vi "Default Settings.vi"() -> (3 "Default Settings":T1={"Log File Base Path"=path "", "Analog Input Channel"="", "Max Value"=0.0, "Min Value"=-5.0})   [LabVIEW 2020, in "Settings Editor.lvlib"]
doc: "_____\nBased on Delacor QMH Project Template 5.0.0.82."
uses:
  Settings Editor.lvlib
  Settings--cluster.ctl
  <vilib>/Utility/sysdir.llb/System Directory Type.ctl
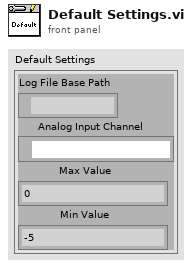
[diagram p1: front panel]
types:
  T1 = typedef "Settings Editor.lvlib/Settings--cluster.ctl" = cluster{"Log File Base Path":path, "Analog Input Channel":refnum<k21>, "Max Value":dbl, "Min Value":dbl}
  T2 = typedef "System Directory Type.ctl" = i32
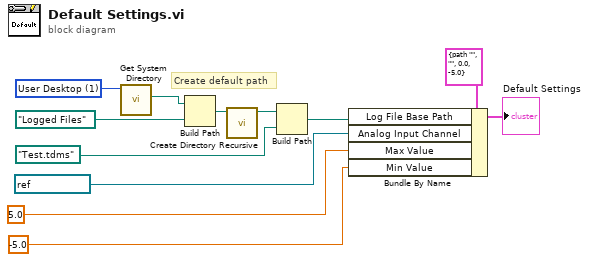
[diagram p0: block diagram]
diagram:
  w12 = T2 1 items=["User Home"=0, "User Desktop"=1, "User Documents"=2, "User Application Data"=3, "User Preferences"=4, "User Temporary"=5, "Public Documents"=6, "Public Application Data"=7, "Public Preferences"=8, "Public Cache"=13, "System Core Libraries"=9, "System Installed Libraries"=10, "Application Files"=11, "Boot Volume Root"=12] ("system directory type")
  # "Create default path"
  n1 = call <vilib>:"Get System Directory.vi"("system directory type"=w12) -> ("system directory"=w11:path)  [unwired: 10 in]
  n2 = Build Path(base path=w11, name or relative path=path "Logged Files") -> (appended path=w10:path)
  n3 = call <vilib>:"Create Directory Recursive.vi"("directory"=w10) -> ("directory copy"=w9:path)  [unwired: 4 in, 2 out]
  n4 = Build Path(base path=w9, name or relative path=path "Test.tdms") -> (appended path=w6:path)
  n5 = Bundle By Name(cluster=T1 {"Log File Base Path"=path "", "Analog Input Channel"="", "Max Value"=0.0, "Min Value"=-5.0} ("Default Settings"), "Log File Base Path"=w6, "Analog Input Channel"=refnum<k21> "Dev0/Ai0", "Max Value"=5.0, "Min Value"=-5.0) -> (→"Default Settings":T1)
